vi "create.mcap_topic.vi"(10 "topic":string) -> (3 "Timestamp Manifest":refnum<class "mcap.lvclass">)   [LabVIEW 2020, in "nominal types.lvlib" / "timestampManifest.lvlib"]
uses:
  mcap/mcap.lvclass
  id/id.lvclass/id.ctl
  mcap/mcap.lvclass/mcap.ctl
  id/id.set.vi
  mcap/mcapChannelLocator.set.vi
  timestampManifest.lvlib
  topic/topic.lvclass
  C:/code/labview-client/lv_src/nominal types/filterTypes/filterTypes.lvclass
  C:/code/labview-client/lv_src/Nominal Client/datasources/payload/payload.lvclass
  C:/code/labview-client/lv_src/nominal types/topic/topic.lvclass
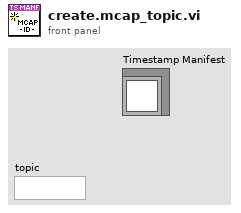
[diagram p1: front panel]
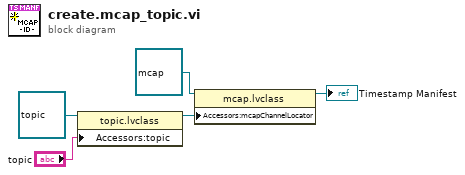
[diagram p0: block diagram]
diagram:
  n1 = property class="topic.lvclass"(reference=refnum<class "topic.lvclass"> refnum ("nominal types.lvlib:channelFilter.lvlib:topic.lvclass"), "Accessors:topic"="topic") -> (reference out=w4:refnum<class "topic.lvclass">)  [unwired: 1 in, 1 out]
  n2 = property class="mcap.lvclass"(reference=refnum<class "mcap.lvclass"> refnum ("nominal types.lvlib:timestampManifest.lvlib:mcap.lvclass"), "Accessors:mcapChannelLocator"=w4) -> (reference out=→"Timestamp Manifest":refnum<class "mcap.lvclass">)  [unwired: 1 in, 1 out]
